vi "readSaveImagesXML.vi"(8 "error in (no error)":errorcluster, 10 "NativeXML in":refnum<class "NativeXML.lvclass">, 11 "PixelflySettings in":refnum<class "PixelflySettings.lvclass">) -> (0 "error out":errorcluster, 2 "NativeXML out":refnum<class "NativeXML.lvclass">, 3 "PixelflySettings out":refnum<class "PixelflySettings.lvclass">)   [LabVIEW 2011, in "Tools.lvlib" / "Settings.lvlib" / "PixelflySettings.lvclass"]
uses:
  PixelflySettings.lvclass
  NativeXML/NativeXML.lvclass
  PixelflySettings.lvclass/PixelflySettings.ctl
  CamaraSettings.lvclass
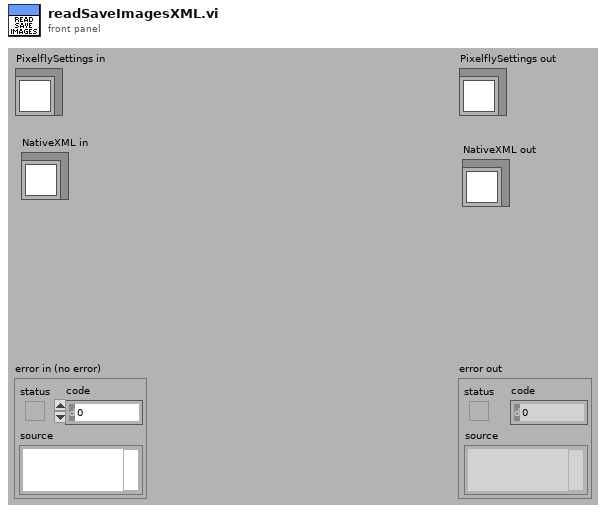
[diagram p1: front panel]
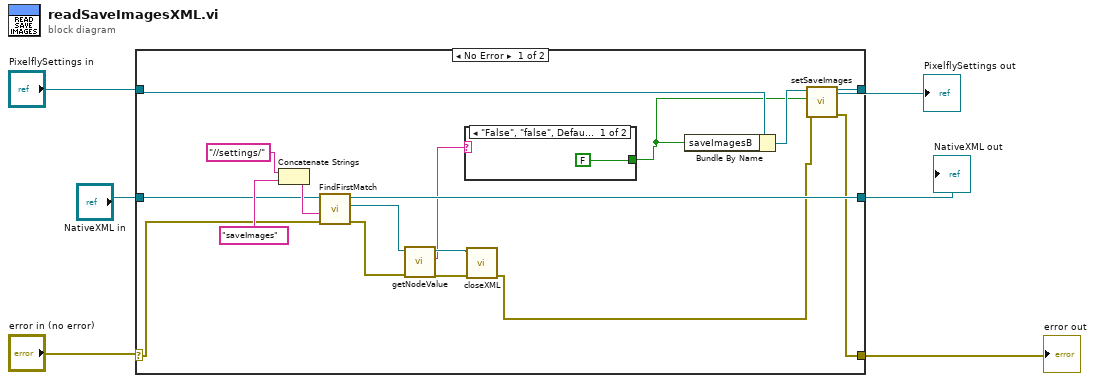
[diagram p0: block diagram]
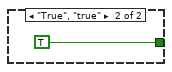
[diagram p2: hidden frame]
diagram:
  n1 = case shown="No Error" "error in (no error)" {
    selector: "error in (no error)" -> [w16 w26]
    tunnel: [w8 w26] -> w5
    tunnel: [w7 w27] -> w4
    tunnel: "PixelflySettings in" -> [w12 w27]
    tunnel: "NativeXML in" -> [w14 w28]
    tunnel: [w19 w28] -> w1
    frame No Error {
      n2 = Concatenate Strings("//settings/" ("searchElementIn"), "saveImages") -> (w15:string)
      n3 = call "FindFirstMatch.vi"("error in (no error)"=w16, "xPath"=w15, "NativeXML in"=w14) -> ("error out"=w17:errorcluster, "NativeXML match"=w18:refnum<class "NativeXML.lvclass">, "NativeXML out"=w19:refnum<class "NativeXML.lvclass">)  [unwired: 6 in]
      n4 = call "getNodeValue.vi"("error in (no error)"=w17, "NativeXML in"=w18) -> ("error out"=w22:errorcluster, "Value"=w13:string, "NativeXML out"=w23:refnum<class "NativeXML.lvclass">)  [unwired: 7 in]
      n5 = case shown="\"False\", \"false\", Default" w13 {
        tunnel: [FALSE TRUE] -> w10
        frame "False", "false", Default {
        }
        frame "True", "true" {
        }
      }
      n6 = call "closeXML.vi"("error in (no error)"=w22, "NativeXML in"=w23) -> ("error out"=w9:errorcluster)  [unwired: 9 in]
      n7 = Bundle By Name(cluster=w12, "saveImagesB"=w10) -> (w11:refnum<class "PixelflySettings.lvclass">)
      n8 = call "setSaveImages.vi"("error in (no error)"=w9, "saveImages"=w10, "CamaraSettings in"=w11) -> ("error out"=w8:errorcluster, "CamaraSettings out"=w7:refnum<class "PixelflySettings.lvclass">)  [unwired: 7 in]
    }
    frame Error {
    }
  }
  "error out" <- w5
  "PixelflySettings out" <- w4
  "NativeXML out" <- w1
